vi "Write Read Data.vi"(0 "Connection ID":refnum<k5>) -> (4 "Connection ID (Dup)":refnum<k5>)   [LabVIEW 2016]
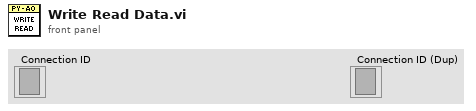
[diagram p1: front panel]
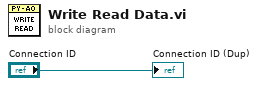
[diagram p0: block diagram]
diagram:
  "Connection ID (Dup)" <- "Connection ID"
